vi "Version 1_Read Output Definitions.vi"(7 "Address (A)":string="A", 8 "error in":errorcluster, 10 "Software Version (optional - wire for speed)":u8, 11 "VISA Session In":refnum<visa-resource-name>="Alicat") -> (0 "error out":errorcluster, 1 "Read-Only Options":T1, 2 "Read/Write Options":T2, 3 "VISA Session Out":refnum<visa-resource-name>)   [LabVIEW 2020]
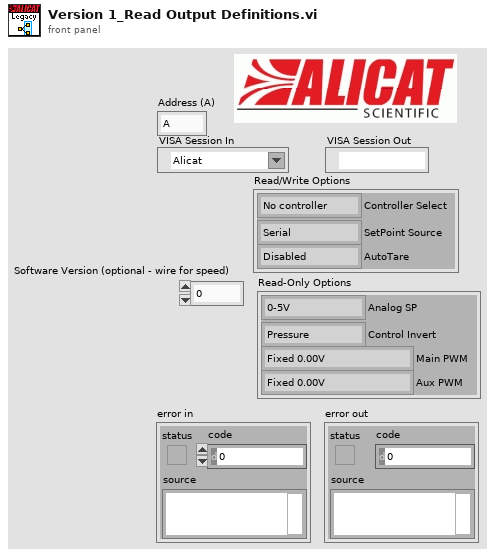
[diagram p1: front panel]
types:
  T1 = cluster{"Analog SP":enum16{"0-5V", "4-20mA"}, "Control Invert":enum16{"Pressure", "Vacuum/BP"}, "Main PWM":enum8{"Fixed 0.00V", "Pressure 0-5V", "Temperature 0-5V", "Volumetric Flow 0-5V", "Mass Flow 0-5V", "Pressure 0-2.5-5V bidir", "Temperature 0-2.5-5V bidir", "Volumetric Flow 0-2.5-5V bidir", "Mass Flow 0-2.5-5V bidir", "Pressure 1-5V", "Temperature 1-5V", "Volumetric Flow 1-5V", "Mass Flow 1-5V", "Reserved(A)", "Reserved(B)", "Fixed 5.12V"}, "Aux PWM":enum8{"Fixed 0.00V", "Pressure 0-5V", "Temperature 0-5V", "Volumetric Flow 0-5V", "Mass Flow 0-5V", "Pressure 0-2.5-5V bidir", "Temperature 0-2.5-5V bidir", "Volumetric Flow 0-2.5-5V bidir", "Mass Flow 0-2.5-5V bidir", "Pressure 1-5V", "Temperature 1-5V", "Volumetric Flow 1-5V", "Mass Flow 1-5V", "Reserved(A)", "Reserved(B)", "Fixed 5.12V"}}
  T2 = cluster{"Controller Select":enum8{"No controller", "Pressure", "Temperature", "Volumetric Flow", "Mass Flow", "Unknown"}, "SetPoint Source":enum8{"Serial", "Local", "Analog", "Unknown"}, "AutoTare":enum16{"Disabled", "Enabled"}}
  T3 = enum8{"No controller", "Pressure", "Temperature", "Volumetric Flow", "Mass Flow", "Unknown"}
  T4 = cluster{"Controller Select":u16, "SetPoint Source":enum8{"Serial", "Local", "Analog", "Unknown"}, "AutoTare":enum16{"Disabled", "Enabled"}}
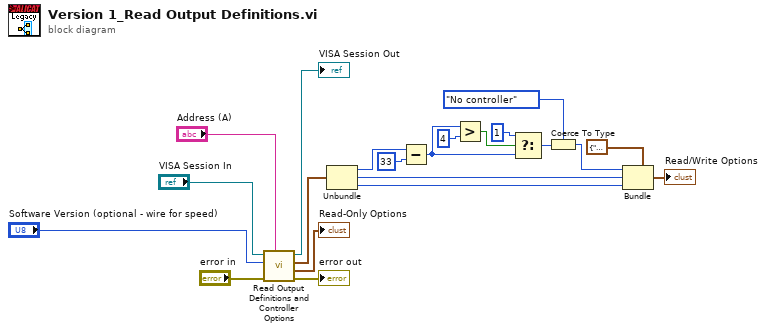
[diagram p0: block diagram]
diagram:
  n1 = call "Read Output Definitions and Controller Options.vi"("Unit ID (A)"="Address (A)", "error in"="error in", "Software Version"="Software Version (optional - wire for speed)", "VISA Session In"="VISA Session In") -> ("error out"=→"error out":errorcluster, "Read-Only Options"=→"Read-Only Options":T1, "Read/Write Options"=w14:T4, "VISA Session Out"=→"VISA Session Out":refnum<visa-resource-name>)  [unwired: 4 in]
  n2 = Unbundle(w14) -> ("Controller Select"=w13:u16, "SetPoint Source"=w2:enum8{"Serial", "Local", "Analog", "Unknown"}, "AutoTare"=w1:enum16{"Disabled", "Enabled"})
  n3 = Subtract(x=w13, y=u16 33) -> (x-y=w9:u16)
  n4 = Greater?(x=w9, y=u16 4) -> (0:w10:bool)
  n5 = Select(t=u16 1, s=w10, f=w9) -> (s? t:f=w4:u16)
  n6 = Coerce To Type(0:w4, 1:T3."No controller" ("Controller Select")) -> (2:w3:T3)
  n7 = Bundle(cluster=T2 {"Controller Select"=enum."No controller", "SetPoint Source"=enum."Serial", "AutoTare"=enum."Disabled"} ("Read/Write Options"), "Controller Select"=w3, "SetPoint Source"=w2, "AutoTare"=w1) -> (→"Read/Write Options":T2)
